vi "Initialize.vi"   [LabVIEW 2019]
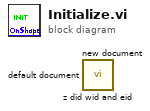
[diagram p0: block diagram]
diagram:
  n1 = call <userlib>:"z did wid and eid.vi"() -> ()  [unwired: 14 in, 2 out]
  n2 = call <userlib>:"new document.vi"() -> ()  [unwired: 13 in, 3 out]
  n3 = call <userlib>:"default document.vi"() -> ()  [unwired: 13 in, 3 out]
